vi "Scroll Panel Into View.vi"(8 "error in (no error)":errorcluster, 9 "Highlight (F)":bool, 10 "Panel Index":i32, 11 "ArrayManager in":refnum<class "ArrayManager.lvclass">) -> (0 "error out":errorcluster, 3 "ArrayManager out":refnum<class "ArrayManager.lvclass">)   [LabVIEW 2020, in "OOPanel.lvlib" / "ArrayManager.lvclass"]
doc: "Sets the scroll such that the panel at the specified panel is fully in view or if it's too big it will be aligned to the top of the view. Optionally highlights the panel after scrolling into view.\n\nIf the panel is off the bottom of the view, the view will be scrolled down so the panel aligns at the bottom of the view. If the panel is off the top of the view, the view will be scrolled up so it aligns to the top of the view. If the panel is already fully in view, the scroll is not changed."
uses:
  ArrayManager.lvclass
  Scroll Into View.ctl
  ArrayManager.lvclass/ArrayManager.ctl
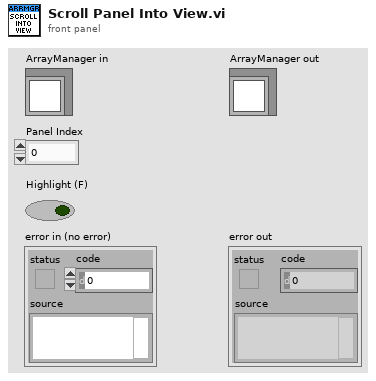
[diagram p1: front panel]
types:
  T1 = typedef "OOPanel.lvlib/ArrayManager.lvclass/Scroll Into View.ctl" = cluster{"Panel Index":i32, "Highlight":bool}
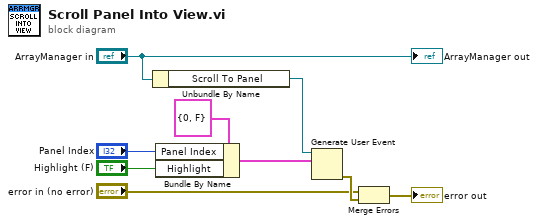
[diagram p0: block diagram]
diagram:
  n1 = Unbundle By Name("ArrayManager in") -> ("Scroll To Panel"=w8:refnum<user-event>)
  n2 = Bundle By Name(cluster=T1 {"Panel Index"=0, "Highlight"=FALSE} ("Scroll Into View"), "Panel Index"="Panel Index", "Highlight"="Highlight (F)") -> (w1:T1)
  n3 = Generate User Event(user event=w8, event data cluster=w1) -> (error out=w7:errorcluster)  [unwired: 2 in, 1 out]
  n4 = Merge Errors("error in (no error)", w7) -> (→"error out":errorcluster)
  "ArrayManager out" <- "ArrayManager in"
